vi "VI Server Launcher23.vi"() -> ()   [LabVIEW 2021]
uses:
  363d3bde-6874-4068-849e-62e045d4c070.vi
  <vilib>/Comparison/Less/Less Functor/Less Functor.lvclass
  <vilib>/Utility/LVLibp/NI_PackedLibraryUtility.lvlib
  CIFUtilities/CIFConfigurationFile/typedef/Location Type.ctl
  CIFUtilities/CIFConfigurationFile/CIF Configuration File.lvlib
panel:
  out "error out":errorcluster
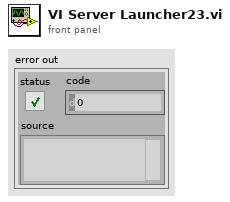
[diagram p1: front panel]
types:
  T1 = enum32{"Invalid", "Standard", "Closed", "Hidden", "Minimized", "Maximized"}
  T2 = typedef "CIF Configuration File.lvlib/Location Type.ctl" = enum16{"Config File", "Manager", "Protos", "Plugins", "UI Plugins", "Logs", "Orchestrations"}
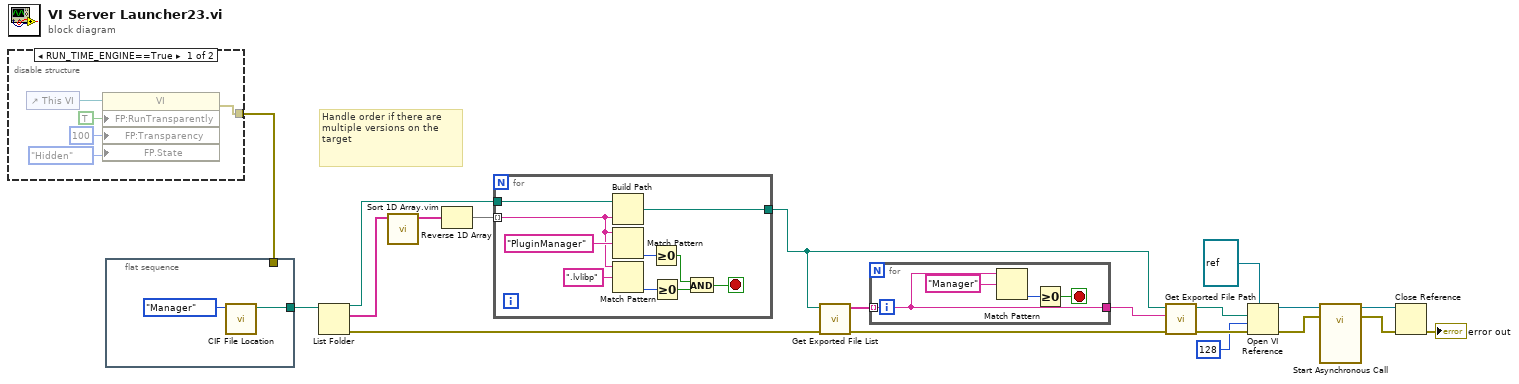
[diagram p0: block diagram]
diagram:
  # "Handle order if there are multiple versions on the target"
  n1 = disable-structure shown="RUN_TIME_ENGINE==True" {
    disable-tunnel: [w24 _] -> w2
    frame condition #0 {
      n2 = control-ref of="This VI"() -> (w25:refnum<vi>)
      n3 = property class="VI"(reference=w25, "FP:RunTransparently"=TRUE ("Front Panel Window:Run VI Transparently"), "FP:Transparency"=u8 100 ("Front Panel Window:Transparency"), "FP.State"=T1."Hidden" ("Front Panel Window:State")) -> (error out=w24:errorcluster)  [unwired: 1 in, 1 out]
    }
    frame condition #1 (active) {
    }
  }
  n4 = flat-sequence {
    tunnel: [w26] -> w1
    tunnel: w2 -> [_]
    frame #0 {
      n5 = call "CIF File Location.vi"("LocationType"=Location_Type."Manager") -> ("Location"=w26:path)  [unwired: 10 in]
    }
  }
  n6 = List Folder(path=w1) -> (path out=w19:path, filenames=w16:string[], error out=w20:errorcluster)  [unwired: 3 in, 1 out]
  n7 = call "Sort 1D Array.vim"("unsorted array"=w16) -> ("sorted array"=w15:string[])  [unwired: 10 in]
  n8 = Reverse 1D Array(array=w15) -> (reversed array=w14:string[])
  n9 = for {
    tunnel: w14 -> [w33] mode=indexing
    tunnel: [w34] -> w17
    tunnel: w19 -> [w35]
    stop <- w28 stop-if-true
    n10 = Build Path(base path=w35, name or relative path=w33) -> (appended path=w34:path)
    n11 = Match Pattern(string=w33, regular expression="PluginManager") -> (offset past match=w37:i32)  [unwired: 1 in, 3 out]
    n12 = Match Pattern(string=w33, regular expression=".lvlibp") -> (offset past match=w31:i32)  [unwired: 1 in, 3 out]
    n13 = Greater Or Equal To 0?(x=w37) -> (x >= 0?=w29:bool)
    n14 = Greater Or Equal To 0?(x=w31) -> (x >= 0?=w30:bool)
    n15 = And(x=w29, y=w30) -> (x .and. y?=w28:bool)
  }
  n16 = call <vilib>:"Get Exported File List.vi"("error in (no error)"=w20, "packed library path"=w17) -> ("error out"=w12:errorcluster, "qualified names"=w13:string[])  [unwired: 7 in, 1 out]
  n17 = for {
    tunnel: w13 -> [w38] mode=indexing
    tunnel: [w38] -> w3
    stop <- w40 stop-if-true
    n18 = Match Pattern(string=w38, regular expression="Manager") -> (offset past match=w41:i32)  [unwired: 1 in, 3 out]
    n19 = Greater Or Equal To 0?(x=w41) -> (x >= 0?=w40:bool)
  }
  n20 = call <vilib>:"Get Exported File Path.vi"("error in (no error)"=w12, "qualified name"=w3, "packed library path"=w17) -> ("error out"=w10:errorcluster, "path"=w11:path)  [unwired: 7 in]
  n21 = Open VI Reference(type specifier VI Refnum (for type only)=refnum<vi> refnum, vi path=w11, options=128, error in (no error)=w10) -> (vi reference=w7:refnum<vi>, error out=w6:errorcluster)  [unwired: 2 in]
  n22 = call-by-ref "Start Asynchronous Call"(reference=w7, error in=w6) -> (reference out=w5:refnum<vi>, error out=w4:errorcluster)  [unwired: 12 in]
  n23 = Close Reference(reference=w5, error in (no error)=w4) -> (error out=→"error out":errorcluster)
